vi "Close.vi"(8 "error in (no error)":errorcluster, 11 "navX - Interface in":refnum<class "navX - Interface.lvclass">) -> (0 "error out":errorcluster, 1 "Timed out?":bool, 3 "navX - Interface out":refnum<class "navX - Interface.lvclass">)   [LabVIEW 2015, in "navX Library v3.lvlib" / "navX - Interface.lvclass"]
uses:
  navX - Interface.lvclass
  navX - Interface.lvclass/navX - Interface.ctl
  navX Registry Cache/navX Registry Cache.lvclass
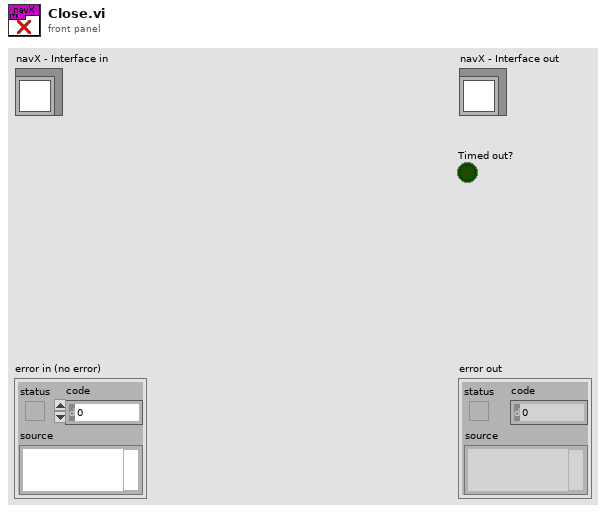
[diagram p1: front panel]
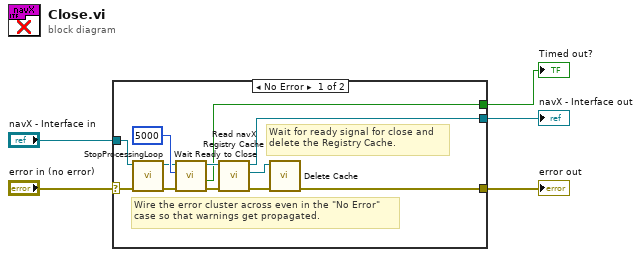
[diagram p0: block diagram]
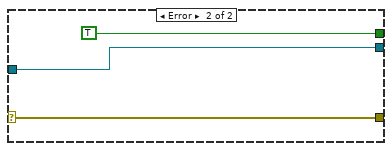
[diagram p2: hidden frame]
diagram:
  n1 = case shown="No Error" "error in (no error)" {
    selector: "error in (no error)" -> [w15 w20]
    tunnel: [w17 w20] -> w4
    tunnel: [w7 w19] -> w2
    tunnel: "navX - Interface in" -> [w16 w19]
    tunnel: [w6 TRUE ("timed out")] -> w1
    frame No Error {
      # "Wire the error cluster across even in the \"No Error\"\ncase so that warnings get propagated."
      # "Wait for ready signal for close and\ndelete the Registry Cache."
      n2 = call "StopProcessingLoop.vi"("error in (no error)"=w15, "navX - Interface in"=w16) -> ("error out"=w14:errorcluster, "navX - Interface out"=w8:refnum<class "navX - Interface.lvclass">)  [unwired: 8 in]
      n3 = call-dynamic "Wait Ready to Close.vi"("error in (no error)"=w14, "ms timeout (-1)"=5000, "navX - Interface in"=w8) -> ("error out"=w10:errorcluster, "timed out"=w6:bool, "navX - Interface out"=w9:refnum<class "navX - Interface.lvclass">)  [unwired: 6 in]
      n4 = call "Read navX Registry Cache.vi"("error in (no error)"=w10, "navX - Interface in"=w9) -> ("error out"=w11:errorcluster, "navX Library v3.lvlib:navX Registry Cache.lvclass"=w12:refnum<class "navX Registry Cache.lvclass">, "navX - Interface out"=w7:refnum<class "navX - Interface.lvclass">)  [unwired: 7 in]
      n5 = call "Delete Cache.vi"("error in (no error)"=w11, "navX Registry Cache in"=w12) -> ("error out"=w17:errorcluster)  [unwired: 7 in, 2 out]
    }
    frame Error {
    }
  }
  "error out" <- w4
  "navX - Interface out" <- w2
  "Timed out?" <- w1
